vi "Msg_WriteLog.vi"(7 "LogType":T1=enum."Manual", 8 "error in":errorcluster, 10 "Text":string, 11 "Base Path":path=path "D:/Vicomm") -> (0 "error out":errorcluster)   [LabVIEW 2019, in "MsgShowAndLog.lvlib"]
uses:
  MsgShowAndLog.lvlib
  Ctrl/LogType.ctl
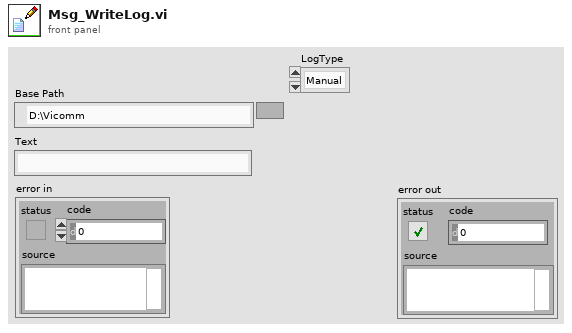
[diagram p1: front panel]
types:
  T1 = typedef "MsgShowAndLog.lvlib/LogType.ctl" = enum16{"Auto", "Manual", "Handshake", "Error"}
  T2 = enum16{"open", "replace", "create", "open or create", "replace or create", "replace or create with confirmation"}
  T3 = typedef "LVDateTimeRec.ctl" = cluster{"fractional second":dbl, "second":i32, "minute":i32, "hour":i32, "day of month":i32, "month":i32, "year":i32, "day of week":i32, "day of year":i32, "DST":i32}
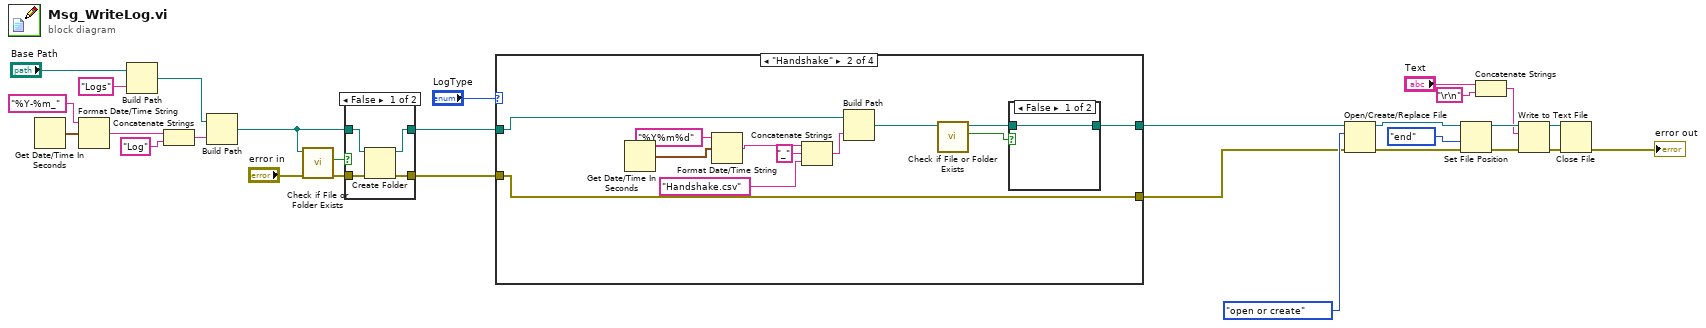
[diagram p0: block diagram]
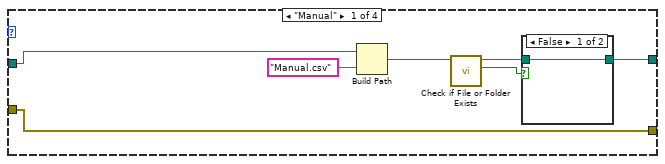
[diagram p2: hidden frame]
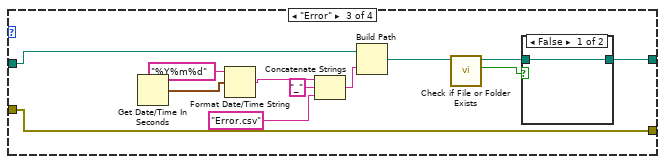
[diagram p5: hidden frame]
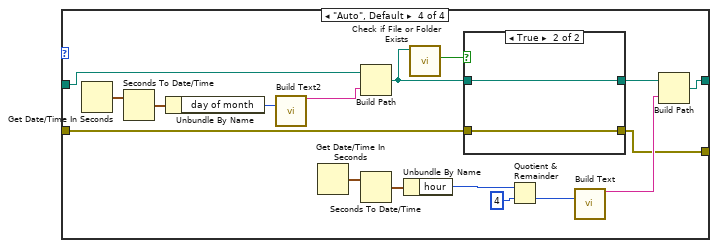
[diagram p7: hidden frame]
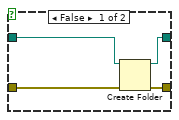
[diagram p8: hidden frame]
diagram:
  n1 = Get Date/Time In Seconds() -> (seconds since 1Jan1904=w26:timestamp)
  n2 = Format Date/Time String(time format string (%c)="%Y-%m_", seconds (now)=w26) -> (date/time string=w24:string)  [unwired: 1 in]
  n3 = Build Path(base path="Base Path", name or relative path="Logs") -> (appended path=w18:path)
  n4 = Concatenate Strings(w24, "Log") -> (w22:string)
  n5 = Build Path(base path=w18, name or relative path=w22) -> (appended path=w28:path)
  n6 = call <vilib>:"Check if File or Folder Exists.vi"("error in (no error)"="error in", "path"=w28) -> ("error out"=w27:errorcluster, "file or folder exists?"=w29:bool)  [unwired: 7 in, 1 out]
  n7 = case shown="False" w29 {
    tunnel: w28 -> [w33 w35]
    tunnel: [w32 w35] -> w14
    tunnel: w27 -> [w31 w34]
    tunnel: [w30 w34] -> w15
    frame False {
      n8 = Create Folder(path (use dialog)=w33, error in=w31) -> (created path=w32:path, error out=w30:errorcluster)  [unwired: 1 in, 1 out]
    }
    frame True {
    }
  }
  n9 = case shown="\"Handshake\"" "LogType" {
    tunnel: w14 -> [w42 w56 w70 w84]
    tunnel: w15 -> [w36 w51 w65 w77]
    tunnel: [w37 w52 w66 w76] -> w16
    tunnel: [w36 w51 w65 w73] -> w1
    frame "Manual" {
      n10 = Build Path(base path=w42, name or relative path="Manual.csv") -> (appended path=w40:path)
      n11 = call <vilib>:"Check if File or Folder Exists.vi"("path"=w40) -> ("file or folder exists?"=w39:bool, "dup path"=w38:path)  [unwired: 8 in, 1 out]
      n12 = case shown="False" w39 {
        tunnel: w38 -> [w43 w44]
        tunnel: [w43 w44] -> w37
        frame False {
        }
        frame True {
        }
      }
    }
    frame "Handshake" {
      n13 = Get Date/Time In Seconds() -> (seconds since 1Jan1904=w50:timestamp)
      n14 = Format Date/Time String(time format string (%c)="%Y%m%d", seconds (now)=w50) -> (date/time string=w46:string)  [unwired: 1 in]
      n15 = Concatenate Strings(w46, "_" ("string"), "Handshake.csv" ("name or relative path")) -> (w48:string)
      n16 = Build Path(base path=w56, name or relative path=w48) -> (appended path=w55:path)
      n17 = call <vilib>:"Check if File or Folder Exists.vi"("path"=w55) -> ("file or folder exists?"=w54:bool, "dup path"=w53:path)  [unwired: 8 in, 1 out]
      n18 = case shown="False" w54 {
        tunnel: w53 -> [w57 w58]
        tunnel: [w57 w58] -> w52
        frame False {
        }
        frame True {
        }
      }
    }
    frame "Error" {
      n19 = Get Date/Time In Seconds() -> (seconds since 1Jan1904=w64:timestamp)
      n20 = Format Date/Time String(time format string (%c)="%Y%m%d", seconds (now)=w64) -> (date/time string=w60:string)  [unwired: 1 in]
      n21 = Concatenate Strings(w60, "_" ("string"), "Error.csv" ("name or relative path")) -> (w62:string)
      n22 = Build Path(base path=w70, name or relative path=w62) -> (appended path=w69:path)
      n23 = call <vilib>:"Check if File or Folder Exists.vi"("path"=w69) -> ("file or folder exists?"=w68:bool, "dup path"=w67:path)  [unwired: 8 in, 1 out]
      n24 = case shown="False" w68 {
        tunnel: w67 -> [w71 w72]
        tunnel: [w71 w72] -> w66
        frame False {
        }
        frame True {
        }
      }
    }
    frame "Auto", Default {
      n25 = Get Date/Time In Seconds() -> (seconds since 1Jan1904=w82:timestamp)
      n26 = Seconds To Date/Time(time stamp (now)=w82) -> (date time rec=w81:T3)  [unwired: 1 in]
      n27 = Unbundle By Name(w81) -> ("day of month"=w83:i32)
      n28 = call "Build Text2"("Date"=w83) -> ("Result"=w80:string)  [unwired: 13 in, 1 out]
      n29 = Get Date/Time In Seconds() -> (seconds since 1Jan1904=w89:timestamp)
      n30 = Build Path(base path=w84, name or relative path=w80) -> (appended path=w75:path)
      n31 = Seconds To Date/Time(time stamp (now)=w89) -> (date time rec=w88:T3)  [unwired: 1 in]
      n32 = Unbundle By Name(w88) -> ("hour"=w86:i32)
      n33 = call <vilib>:"Check if File or Folder Exists.vi"("path"=w75) -> ("file or folder exists?"=w74:bool)  [unwired: 8 in, 2 out]
      n34 = case shown="True" w74 {
        tunnel: w75 -> [w93 w95]
        tunnel: [w92 w95] -> w79
        tunnel: w77 -> [w91 w94]
        tunnel: [w90 w94] -> w73
        frame False {
          n35 = Create Folder(path (use dialog)=w93, error in=w91) -> (created path=w92:path, error out=w90:errorcluster)  [unwired: 1 in, 1 out]
        }
        frame True {
        }
      }
      n36 = Quotient & Remainder(x=w86, y=4) -> (floor(x/y)=w85:i32)  [unwired: 1 out]
      n37 = call "Build Text"("Time"=w85) -> ("Result"=w78:string)  [unwired: 13 in, 1 out]
      n38 = Build Path(base path=w79, name or relative path=w78) -> (appended path=w76:path)
    }
  }
  n39 = Open/Create/Replace File(file path (use dialog)=w16, error in=w1, operation (0:open)=T2."open or create") -> (refnum out=w12:refnum<file>, error out=w10:errorcluster)  [unwired: 3 in, 1 out]
  n40 = Set File Position(refnum=w12, from (0:start)=enum16{"start", "end", "current"}."end", error in=w10) -> (refnum out=w8:refnum<file>, error out=w9:errorcluster)  [unwired: 1 in]
  n41 = Concatenate Strings("Text", "\r\n") -> (w5:string)
  n42 = Write to Text File(file (use dialog)=w8, text=w5, error in=w9) -> (refnum out=w7:refnum<file>, error out=w6:errorcluster)  [unwired: 1 in, 1 out]
  n43 = Close File(refnum=w7, error in=w6) -> (error out=→"error out":errorcluster)  [unwired: 1 out]
